vi "Stopping.vi"(6 "Teller":T1 {"Absolute Time" format="%<%x %.3X>T"}, 8 "Error in":errorcluster, 11 "Base Actor in":refnum<class "Base Actor.lvclass">) -> (0 "Error out":errorcluster, 3 "Base Actor out":refnum<class "Base Actor.lvclass">)   [LabVIEW 2020, in "jettl.lvlib" / "Base jettl Actor.lvlib" / "Base Actor.lvlib" / "Base Actor.lvclass"]
doc: "jettl 6.12.1.94\nNathan Davis - Nathan Davis\nCopyright (c) 2026, Nathan Davis\nMIT"
uses:
  Base Actor.lvclass
  C:/git/jettl/src/jettl/jettl/Actor/Actor.lvclass
  Teller Metadata/Teller Metadata.lvclass
  Base Actor.lvclass/Base Actor.ctl
  C:/git/jettl/src/jettl/jettl/Base jettl Actor/Base Actor/Base Actor/Base Actor.lvclass
  C:/git/jettl/src/jettl/jettl/Start jettl Msg/Start jettl Msg/Start jettl Msg.lvclass
  C:/git/jettl/src/jettl/jettl/Stop jettl Msg/Stop jettl Msg/Stop jettl Msg.lvclass
  C:/git/jettl/src/jettl/jettl/Stopped jettl Msg/Stopped jettl Msg/Stopped jettl Msg.lvclass
  C:/git/jettl/src/jettl/jettl/Stopping jettl Msg/Stopping jettl Msg/Stopping jettl Msg.lvclass
  Stop jettl Msg/Stop/Stop.lvlib
  jettl.lvlib
  Actor Specific/Actor Specific.lvlib
  Stop jettl Msg/Stop/Tell Self.vi
  Actor Specific/Read Lifetime.vi
  Relation.ctl
  Teller.ctl
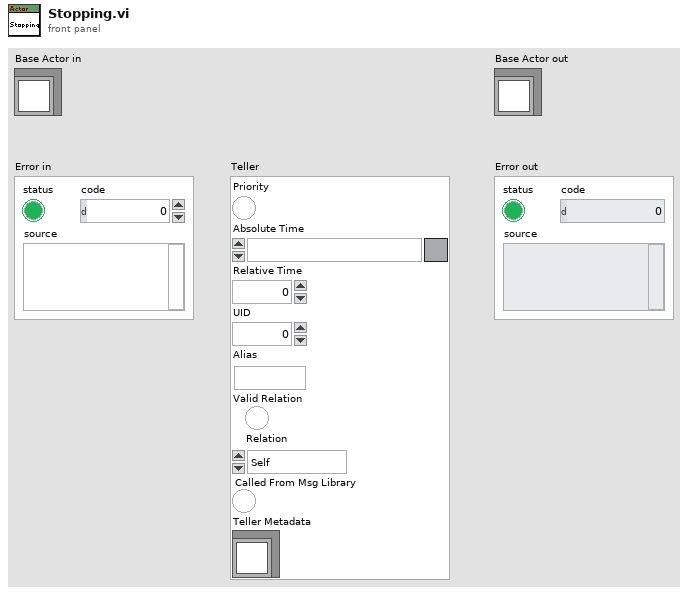
[diagram p1: front panel]
types:
  T1 = typedef "jettl.lvlib/Teller.ctl" = cluster{"Priority":bool, "Absolute Time":timestamp, "Relative Time":dbl, "UID":i32, "Alias":string, "Valid Relation":bool, "Relation":T2, "Called From Msg Library":bool, "Teller Metadata":refnum<class "Teller Metadata.lvclass">}
  T2 = typedef "jettl.lvlib/Relation.ctl" = enum16{"Self", "Parent", "Child"}
  T3 = typedef "jettl.lvlib/Lifetime.ctl" = enum16{"Init", "Spawn", "Setup", "Teardown Before Running", "Running", "Stop Called", "Stopping With Children", "Stopping Without Children", "Teardown After Running", "Stopped"}
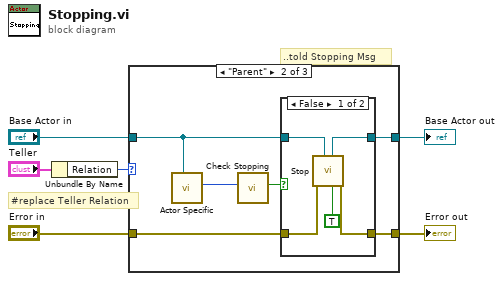
[diagram p0: block diagram]
diagram:
  # "#replace Teller Relation"
  # "..told Stopping Msg"
  n1 = Unbundle By Name("Teller") -> ("Relation"=w1:T2)
  n2 = case shown="\"Parent\"" w1 {
    tunnel: "Base Actor in" -> [w8 w10 w23]
    tunnel: [w8 w14 w23] -> w5
    tunnel: "Error in" -> [w7 w13 w22]
    tunnel: [w7 w12 w22] -> w3
    frame "Self" {
      # "Case will not fundamentally execute"
    }
    frame "Parent" {
      n3 = call-poly "Actor Specific.vi"("Actor in"=w10) -> ("Lifetime"=w9:T3)  [unwired: 10 in]
      n4 = call "Check Stopping.vi"("Lifetime"=w9) -> ("Stopping"=w11:bool)  [unwired: 10 in]
      n5 = case shown="False" w11 {
        tunnel: [w19 w21] -> w14
        tunnel: w13 -> [w18 w20]
        tunnel: [w17 w20] -> w12
        tunnel: w10 -> [w16 w21]
        frame False {
          n6 = call-poly "Stop.vi"("Priority"=TRUE, "Actor in"=w16, "Error in"=w18) -> ("Error out"=w17:errorcluster, "Actor out"=w19:refnum<class "Base Actor.lvclass">)  [unwired: 7 in]
        }
        frame True {
        }
      }
    }
    frame "Child" {
      # "Case will not fundamentally execute"
    }
  }
  "Base Actor out" <- w5
  "Error out" <- w3
